vi "ProcessTraceData.vi"(6 "BaselineRate":dbl=0.01 min=0.0 max=1.0, 7 "decimating factor":i32=10, 8 "Space":i32, 9 "NumPoints":i32, 10 "NumChans":i32, 11 "Data":i32[](array[numeric])) -> (3 "Waveforms":waveform(dbl)[](array[waveform]))   [LabVIEW 2012]
uses:
  <vilib>/Analysis/2dsp.llb/Decimate (continuous, DBL).vi
  <vilib>/Analysis/baseanly.llb/Mean (DBL).vi
  <vilib>/Analysis/NI_AALPro.lvlib
  <vilib>/Analysis/NI_AALBase.lvlib
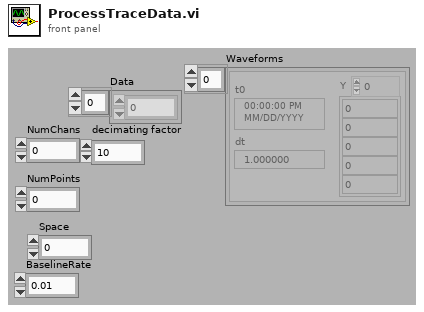
[diagram p1: front panel]
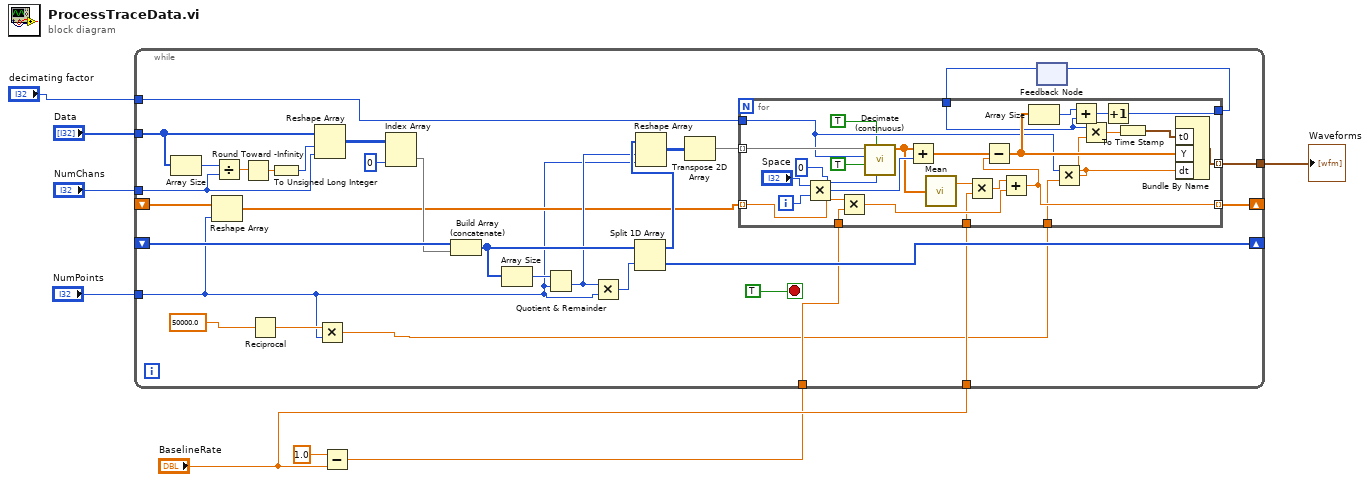
[diagram p0: block diagram]
diagram:
  n1 = Subtract(x=1.0, y="BaselineRate") -> (x-y=w2:dbl)
  n2 = while {
    tunnel: "NumChans" -> [w13]
    shift-right: [w28] -> _
    shift-left: _ -> [w34]
    tunnel: "NumPoints" -> [w12]
    tunnel: "Data" -> [w26]
    tunnel: [w23] -> w5
    shift-right: [w19] -> _
    shift-left: _ -> [w16]
    tunnel: "BaselineRate" -> [w18]
    tunnel: w2 -> [w17]
    tunnel: "decimating factor" -> [w14]
    stop <- TRUE stop-if-true
    n3 = Array Size(array=w26) -> (size(s)=w40:i32)
    n4 = Reshape Array(w16, w12) -> (w15:dbl[])
    n5 = Divide(x=w40, y=w13) -> (x/y=w39:dbl)
    n6 = Round Toward -Infinity(1:w39) -> (0:w38:dbl)
    n7 = Reciprocal(x=50000.0) -> (1/x=w20:dbl)
    n8 = To Unsigned Long Integer(number=w38) -> (unsigned 32bit integer=w37:u32)
    n9 = Reshape Array(w26, w37, w13) -> (w36:i32[][])
    n10 = Multiply(x=w20, y=w12) -> (x*y=w9:dbl)
    n11 = Index Array(array=w36, index (col)=0 ("index (row)")) -> (element=w33:i32[])  [unwired: 1 in]
    n12 = Build Array (concatenate)(w34, w33) -> (w31:i32[])
    n13 = Array Size(array=w31) -> (size(s)=w32:i32)
    n14 = Quotient & Remainder(x=w32, y=w12) -> (floor(x/y)=w22:i32)  [unwired: 1 out]
    n15 = Multiply(x=w22, y=w12) -> (x*y=w30:i32)
    n16 = Split 1D Array(array=w31, index=w30) -> (first subarray=w29:i32[], second subarray=w28:i32[])
    n17 = Reshape Array(w29, w22, w12) -> (w25:i32[][])
    n18 = Transpose 2D Array(2D array=w25) -> (transposed array=w24:i32[][])
    n19 = feedback #1() -> (w10:i32)  [unwired: 1 in]
    n20 = for {
      tunnel: w24 -> [w51] mode=indexing
      tunnel: w14 -> [w44]
      tunnel: w9 -> [w46]
      tunnel: [w62] -> w23 mode=indexing
      tunnel: [w53] -> w19 mode=indexing
      tunnel: w15 -> [w58] mode=indexing
      tunnel: w18 -> [w56]
      tunnel: w17 -> [w55]
      tunnel: [w42] -> w11
      tunnel: w10 -> [w48]
      i -> [w67]
      n21 = Multiply(x="Space", y=w67) -> (x*y=w65:i32)
      n22 = Multiply(x=w58, y=w55) -> (x*y=w57:dbl)
      n23 = call-poly <vilib>:"Decimate (continuous).vi"("start index"=0, "reset"=TRUE, "averaging"=TRUE, "decimating factor"=w44, "X"=w51) -> ("Decimated Array"=w61:dbl[])  [unwired: 5 in, 1 out]
      n24 = Add(x=w61, y=w65) -> (x+y=w54:dbl[])
      n25 = call-poly <vilib>:"Mean.vi"("X"=w61) -> ("mean"=w60:dbl)  [unwired: 1 out]
      n26 = Multiply(x=w60, y=w56) -> (x*y=w59:dbl)
      n27 = Add(x=w59, y=w57) -> (x+y=w53:dbl)
      n28 = Subtract(x=w54, y=w53) -> (x-y=w52:dbl[])
      n29 = Array Size(array=w52) -> (size(s)=w49:i32)
      n30 = Multiply(x=w44, y=w46) -> (x*y=w45:dbl)
      n31 = Add(x=w49, y=w48) -> (x+y=w43:i32)
      n32 = Multiply(x=w48, y=w45) -> (x*y=w50:dbl)
      n33 = Increment(x=w43) -> (x+1=w42:i32)
      n34 = To Time Stamp(1:w50) -> (0:w47:timestamp)
      n35 = Bundle By Name("t0"=w47, "Y"=w52, "dt"=w45) -> (w62:waveform(dbl))  [unwired: 1 in]
    }
    n36 = feedback-in #1(w11) -> ()
  }
  "Waveforms" <- w5
